vi "Variant Pop Up.vi"(8 "error in (no error)":errorcluster, 11 "Variant":variant) -> (0 "error out":errorcluster)   [LabVIEW 2016, in "SLL Debug.lvlib"]
doc: "Takes a variant input and converts to JSON and displays it as a blocking pop up, with option of suppressing further pop ups."
uses:
  SLL Debug.lvlib
  <vilib>/addons/_JKI.lib/Serialization/JSON/JKI JSON Serialization.lvlib
panel:
  out "Call Chain (Inner Most Caller at Top)":string
  in  "OK":bool
  in  "Suppress Further Pop Ups?":bool
  out "Data Display":string
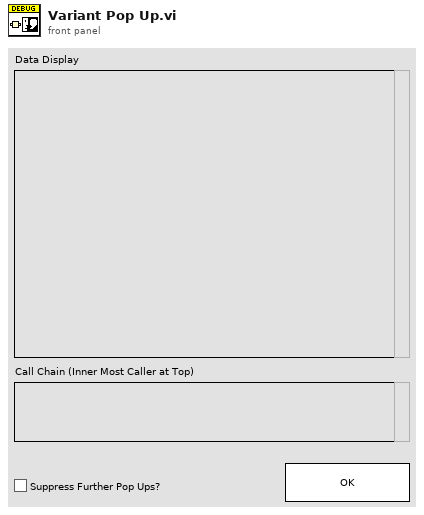
[diagram p1: front panel]
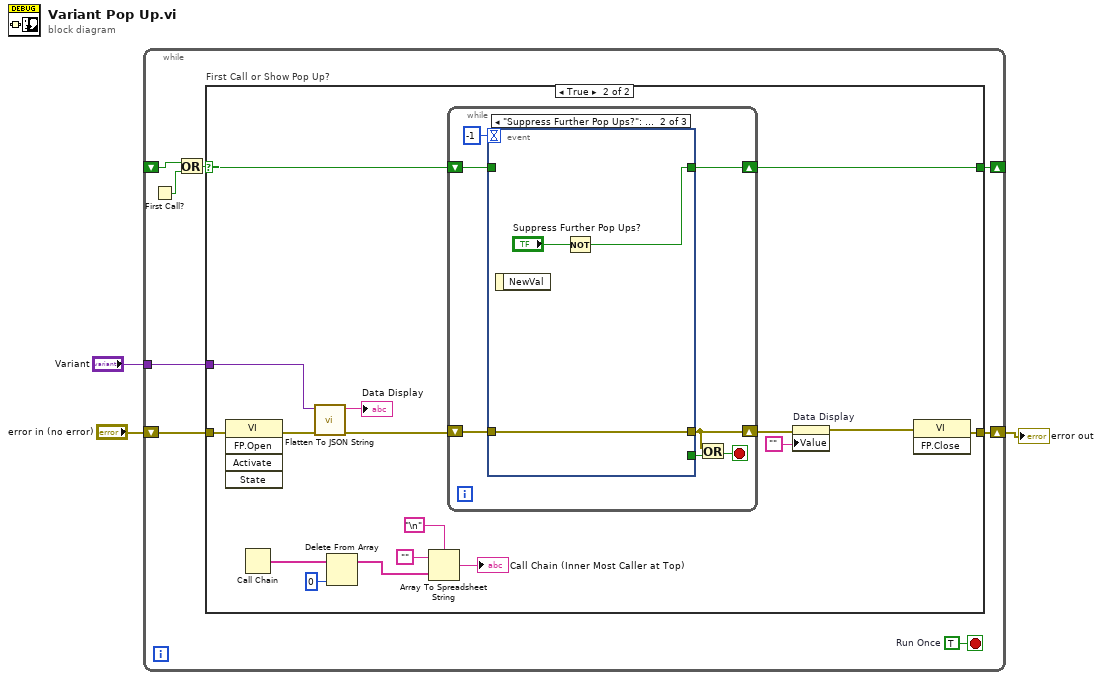
[diagram p0: block diagram]
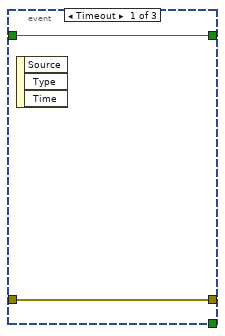
[diagram p3: hidden frame]
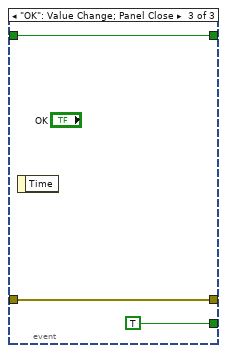
[diagram p4: hidden frame]
diagram:
  n1 = while {
    shift-right: [w8] -> _
    shift-left: _ -> [w7]
    shift-right: [w5] -> w3
    shift-left: "error in (no error)" -> [w6]
    tunnel: "Variant" -> [w4]
    stop <- w11 stop-if-true
    w11 = TRUE  # Run Once
    n2 = First Call?() -> (First Call?: T/F=w10:bool)
    n3 = Or(x=w7, y=w10) -> (x .or. y?=w9:bool)
    n4 = case "First Call or Show Pop Up?" shown="True" w9 {
      selector: w9 -> [w13 w30]
      tunnel: [w13 w29] -> w8
      tunnel: w6 -> [w12 w28]
      tunnel: [w12 w25] -> w5
      tunnel: w4 -> [_ w26]
      frame False {
      }
      frame True {
        n5 = invoke class="VI" method="FP.Open"(error in=w28) -> (error out=w27:errorcluster)  [unwired: 4 in, 4 out]
        n6 = Call Chain() -> (call chain=w16:string[])
        n7 = call <vilib>:"Flatten To JSON String.vi"("error in (no error)"=w27, "Variant"=w26) -> ("error out"=w24:errorcluster, "JSON String"=→"Data Display":string)  [unwired: 8 in]
        n8 = Delete From Array(array=w16, index=0) -> (array with subset deleted=w14:string[])  [unwired: 1 in, 1 out]
        n9 = Array To Spreadsheet String(delimiter (Tab)="\n", array=w14, 3:"") -> (spreadsheet string=→"Call Chain (Inner Most Caller at Top)":string)
        n10 = while {
          shift-right: [w35] -> w29
          shift-left: w30 -> [w36]
          shift-right: [w31] -> w22
          shift-left: w24 -> [w34]
          stop <- w32 stop-if-true
          n11 = event shown="[1] \"Suppress Further Pop Ups?\": Value Change" {
            selector: _ -> [_ _ _]
            dyn-events: _ -> [_ _ _]
            timeout: -1 -> [_ _ _]
            tunnel: [w39 w41 w45] -> w35
            tunnel: w36 -> [w39 _ w45]
            tunnel: [_ _ TRUE] -> w33
            tunnel: w34 -> [w38 w40 w43]
            tunnel: [w38 w40 w43] -> w31
            event Timeout {
              n12 = event-data() -> ()  [unwired: 1 in, 3 out]
            }
            event "Suppress Further Pop Ups?": Value Change {
              n13 = event-data() -> ()  [unwired: 1 in, 1 out]
              n14 = Not(x="Suppress Further Pop Ups?") -> (.not. x?=w41:bool)
            }
            event "OK": Value Change; Panel Close {
              n15 = event-data() -> ()  [unwired: 1 in, 1 out]
            }
          }
          n16 = Or(x=w31, y=w33) -> (x .or. y?=w32:bool)
        }
        n17 = property on="Data Display" class="Str"(error in=w22, "Value"="") -> (error out=w21:errorcluster)  [unwired: 1 in, 1 out]
        n18 = invoke class="VI" method="FP.Close"(error in=w21) -> (error out=w25:errorcluster)  [unwired: 2 in, 2 out]
      }
    }
  }
  "error out" <- w3
